vi "API.vi"(8 "error in (no error)":errorcluster, 11 "BasicEventLogger in":refnum<class "BasicEventLogger.lvclass">) -> (0 "error out":errorcluster, 2 "API":refnum<class "API.lvclass">, 3 "BasicEventLogger out":refnum<class "BasicEventLogger.lvclass">)   [LabVIEW 2020, in "Volatus.lvlib" / "BasicEventLogger.lvclass"]
uses:
  BasicEventLogger.lvclass
  C:/Program Files (x86)/National Instruments/LabVIEW 2020/vi.lib/ActorFramework/Actor/Actor.lvclass
  API/API.lvclass
  <vilib>/ActorFramework/Actor/Actor.lvclass/Actor.ctl
  <vilib>/ActorFramework/Message Enqueuer/Message Enqueuer.lvclass/Message Enqueuer.ctl
  <vilib>/ActorFramework/Message Enqueuer/Init from Existing Queue.vi
  Event API/EventAPI.lvclass
  C:/dev/lv20CE/relink/lv-volatus/Volatus/API/API.lvclass
  <vilib>/ActorFramework/Message Enqueuer/Message Enqueuer.lvclass
  BasicEventLogger.lvclass/BasicEventLogger.ctl
  <vilib>/ActorFramework/Actor/Actor.lvclass
  C:/dev/lv20CE/relink/lv-volatus/Volatus/Task/Task.lvclass
  C:/dev/lv20CE/relink/lv-volatus/Volatus/VectoMessageHandler/VectoMessageHandler.lvclass
  C:/dev/lv20CE/relink/lv-volatus/Volatus/TaskStateHandler/TaskStateHandler.lvclass
  C:/dev/lv20CE/relink/lv-volatus/Volatus/BasicEventLogger/BasicEventLogger.lvclass
  C:/dev/lv20CE/relink/lv-volatus/Volatus/API Provider/API Provider.lvclass
  C:/dev/lv20CE/relink/lv-volatus/Volatus/Event API/EventAPI.lvclass
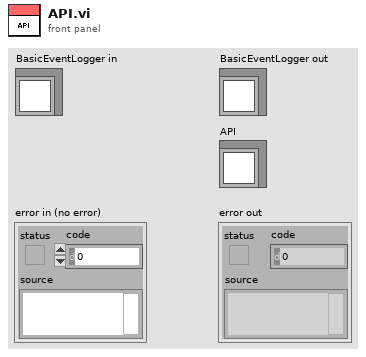
[diagram p1: front panel]
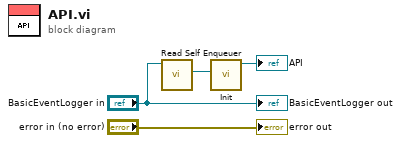
[diagram p0: block diagram]
diagram:
  n1 = call <vilib>:"Read Self Enqueuer.vi"("Actor"="BasicEventLogger in") -> ("Self Enqueuer"=w2:refnum<class "Message Enqueuer.lvclass">)  [unwired: 10 in]
  n2 = call "Init.vi"("EnQr"=w2) -> ("Event API out"=→"API":refnum<class "EventAPI.lvclass">)  [unwired: 9 in, 1 out]
  "error out" <- "error in (no error)"
  "BasicEventLogger out" <- "BasicEventLogger in"
